vi "Delete Signal DVR.vi"(8 "error in (no error)":errorcluster, 11 "Signal DVR in":refnum<data-value>) -> (0 "error out":errorcluster, 3 "Signal out":refnum<class "Signal.lvclass">)   [LabVIEW 2012, in "MDSplus.lvlib" / "Signal.lvclass"]
uses:
  <vilib>/MDSplus/Classes/Data_Class/Compound_Class/Signal_Class/Signal.lvclass
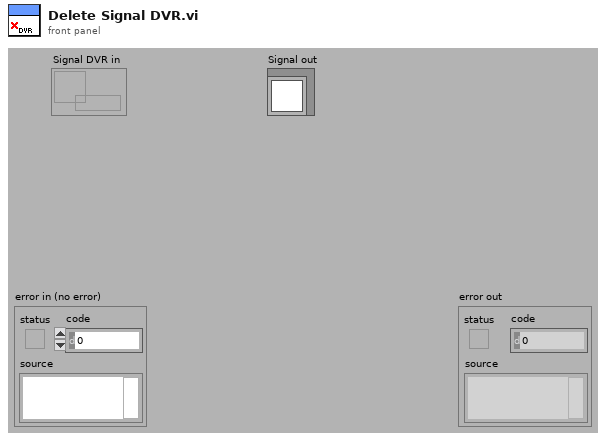
[diagram p1: front panel]
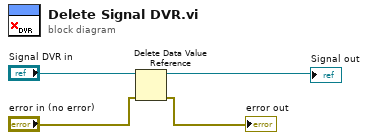
[diagram p0: block diagram]
diagram:
  n1 = Delete Data Value Reference(data value reference="Signal DVR in", error in="error in (no error)") -> (data value=→"Signal out":refnum<class "Signal.lvclass">, error out=→"error out":errorcluster)
